vi "References.vi"() -> ()   [LabVIEW 2018]
uses:
  VisionLibrariesXimea/xiLib/xiLIB_64bit/xiLIB/xiCamLib/xiCam/PRM/IMG_FORMAT/IMG_DATA_FORMAT.ctl
panel:
  in  "pixel size (um)":dbl=3.9
  in  "wavelength (nm)":dbl=780.0
  in  "IMG_FORMAT":T1
  in  "exposure (us)":dbl=100.0
  in  "Main only":dbl[][](array[numeric])
  in  "Ref only":dbl[][](array[numeric])
  in  "Background":dbl[][](array[numeric])
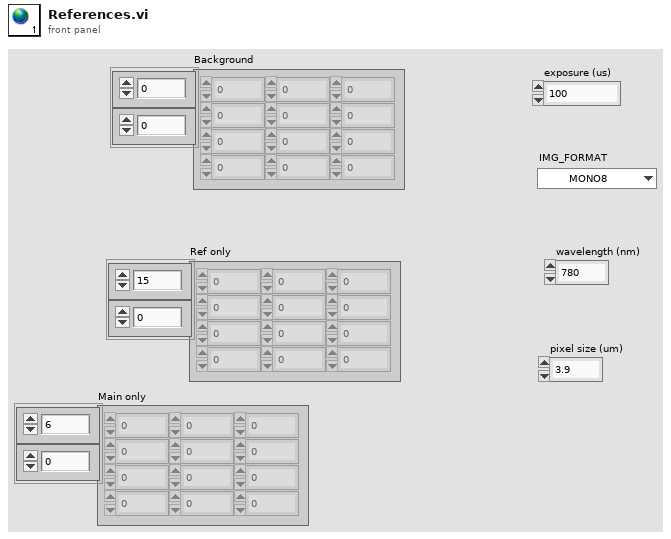
[diagram p1: front panel]
types:
  T1 = typedef "IMG_DATA_FORMAT.ctl" = enum16{"MONO8", "MONO16", "RGB24", "RGB32", "RGBPLANAR", "RAW8", "RAW16"}
diagram:
